vi "PH_PPMA_PowerUnit.PC_StateIgni.vi"(0 "i ref in":refnum<vi>, 3 "Ignitron Status":T1=2 caption="Enabling State" items=["no info", "off/false/out", "on/true/in", "Failure", "Alarm", "Status 1", "Status 2", "Status 3"], 4 "not linked?":bool, 5 "error in (no error)":errorcluster) -> (14 "i ref out":refnum<vi>, 19 "error out":errorcluster)   [LabVIEW 2014, in "PH_PPMA_PowerUnit.lvlib"]
doc: "This VI writes the Ignitron Tag values to own attributes, calculates the state of the device and sets the GUI object."
uses:
  PH_PPMA_PowerUnit.lvlib
  PH_Basics/PH_StatusHandler/PH_StatusHandler.Status.ctl
  PH_Basics/PH_Common/PH_Common.lvlib
  PH_Devices/PH_Beckhoff_PP_PU/PH_Beckhoff_PP_PU.lvlib
  PH_Basics/PH_PowerUnit_BaseClass/PH_PowerUnit_BaseClass.lvlib
  PH_Basics/PH_StatusHandler/PH_StatusHandler.lvlib
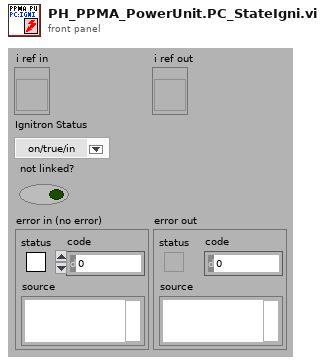
[diagram p1: front panel]
types:
  T1 = typedef "PH_StatusHandler.lvlib/PH_StatusHandler.Status.ctl" = i16
  T2 = typedef "PH_PPMA_PowerUnit.lvlib/PH_PPMA_PowerUnit.i attribute.ctl" = cluster{"GUI Refs":cluster{"Rods":refnum<vi>, "Ignitron":refnum<vi>, "Rossrelais":refnum<vi>, "Set Voltage":refnum<vi>, "PSU":refnum<vi>, "EOC":refnum<vi>, "Trigger":refnum<vi>}, "Rods":T3, "PSU":T4, "Ross Relais":T5, "Ignitron":T6, "Trigger":cluster{"State Device":T1, "linked?":bool}, "Timing Settings":cluster{"Prdc Fast?":bool, "Default Value Periodic Interval":i32, "Mercury on since":dbl, "Warm up Time Mercury [s]":dbl}, "Set Voltage [V]":dbl}
  T3 = typedef "PH_PPMA_PowerUnit.lvlib/PH_PPMA_PowerUnit.Rods Attributes.ctl" = cluster{"Instancename":string, "Device Status":T1, "linked?":bool}
  T4 = typedef "PH_PP_Common.lvlib/PH_PP_Common.PSU Attributes.ctl" = cluster{"lower limit [V]":dbl, "upper limit [V]":dbl, "Voltage set":bool, "State Device":T1, "linked?":bool}
  T5 = typedef "PH_PP_Common.lvlib/PH_PP_Common.Ross Relais Attributes.ctl" = cluster{"State Device":T1, "linked?":bool}
  T6 = typedef "PH_PP_Common.lvlib/PH_PP_Common.Ignitron Attributes.ctl" = cluster{"State Device":T1, "linked?":bool}
  T7 = typedef "PH_PowerUnit_BaseClass.lvlib/PH_PowerUnit_BaseClass.i attribute.ctl" = cluster{"Constructor finished":bool, "PU":cluster{"In use":bool, "Service ID in use":i32, "GUI Ref":refnum<vi>}, "Enabling":cluster{"State":T8, "GUI Ref":refnum<vi>}, "Timing":cluster{"Last Shot":dbl, "Time between Shots [Sec]":dbl, "Waiting Time over?":bool, "Service ID Waiting Time":i32, "GUI Ref":refnum<vi>, "Instance":cluster{"Status":T1, "linked?":bool, "GUI Ref":refnum<vi>}}, "Sequencer":cluster{"SM State":string, "GUI Ref":refnum<vi>, "linked":bool}, "Subscribed Trendmssgs":cluster{"Tagname":string, "Status":T1, "linked?":bool, "Shot Condition":T1, "GUI Ref":refnum<vi>}[], "PP PU":T9, "Default Voltage (V)":dbl, "GUI Refs":T10, "PSDB data":cluster{"Shot Voltage [V]":dbl, "State TO SM":T11, "Write 2 early":bool}, "State TO SM":T11}
  T8 = typedef "PH_SystemInformation.lvlib/PH_SystemInformationEnabling State.ctl" = i32
  T9 = typedef "PH_PP_Common.lvlib/PH_PP_Common.PUs.ctl" = enum16{"no Info", "PA-19mm-1", "PA-19mm-2", "PA-45mm-PILC", "PA-45mm-MAIN", "MA-PU-1", "MA-PU-2", "MA-PU-3", "MA-PU-4", "MA-PU-5", "MA-PU-6", "MA-FR", "MA-PILC", "PA-45mm-DP"}
  T10 = typedef "PH_PowerUnit_BaseClass.lvlib/PH_PowerUnit_BaseClass.GUI Refs.ctl" = cluster{"Delete Inst":refnum<vi>, "State TO SM":refnum<vi>, "State SM":refnum<vi>, "Fire":refnum<vi>}
  T11 = typedef "PH_PowerUnit_BaseClass.lvlib/PH_PowerUnit_BaseClass.SM States.ctl" = enum16{".", "Stand by", "Switch PU on", "Configure", "Set Default Voltage", "Set STANDBY", "Set READY", "Wait for Shot Cmd", "Open Dump Rods", "Open Ross Relais", "Close Ross Relais", "Switch PSU on", "Switch PSU off", "Charge", "Switch GD Channel on", "Close Dump Rods", "Rods-TO", "RR-TO", "PSU-TO", "Trigger-TO"}
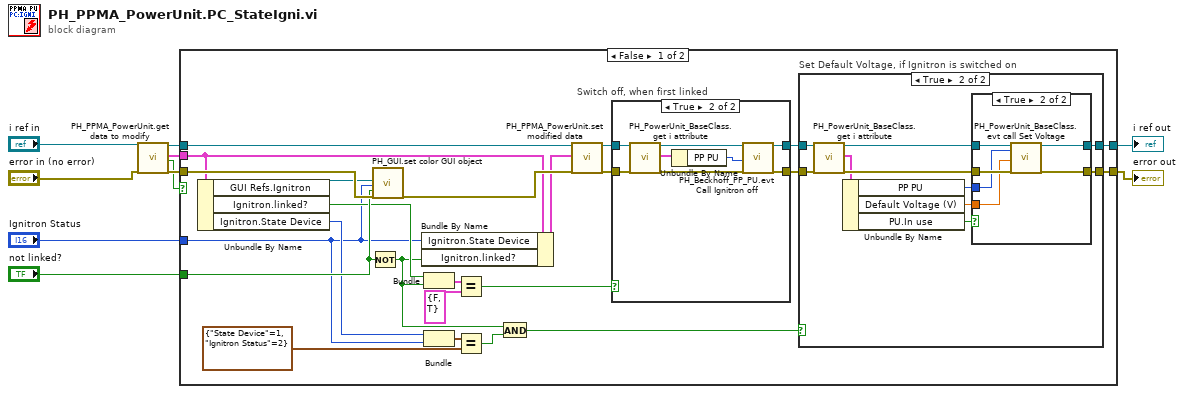
[diagram p0: block diagram]
diagram:
  n1 = call "PH_PPMA_PowerUnit.get data to modify.vi"("i ref in"="i ref in", "error in (no error)"="error in (no error)") -> ("i ref out"=w10:refnum<vi>, "i attribute"=w8:T2, "timed out"=w7:bool, "error out"=w9:errorcluster)  [unwired: 14 in]
  n2 = case shown="False" w7 {
    tunnel: w10 -> [w34 w66]
    tunnel: [w21 w66] -> w4
    tunnel: w9 -> [w33 w65]
    tunnel: [w19 w65] -> w3
    tunnel: w8 -> [w29 _]
    tunnel: "Ignitron Status" -> [w16 _]
    tunnel: "not linked?" -> [w28 _]
    frame False {
      n3 = Unbundle By Name(w29) -> ("GUI Refs.Ignitron"=w30:refnum<vi>, "Ignitron.linked?"=w27:bool, "Ignitron.State Device"=w17:T1)
      n4 = Not(x=w28) -> (.not. x?=w11:bool)
      n5 = call "PH_GUI.set color GUI object.vi"("GUI object Ref"=w30, "State"=w16, "Blinking? (false)"=w28, "error in (no error)"=w33) -> ("error out"=w32:errorcluster)  [unwired: 15 in]
      n6 = Bundle By Name(cluster=w29, "Ignitron.State Device"=w16, "Ignitron.linked?"=w11) -> (w31:T2)
      n7 = Bundle("linked?"=w27, w11) -> (w26:cluster{"linked?":bool, bool})  [unwired: 1 in]
      n8 = Bundle("State Device"=w17, "Ignitron Status"=w16) -> (w15:cluster{"State Device":T1, "Ignitron Status":T1})  [unwired: 1 in]
      n9 = Equal?(x=w26, y=cluster{"linked?":bool, bool} {"linked?"=FALSE, TRUE}) -> (x = y?=w22:bool)
      n10 = Equal?(x=w15, y=cluster{"State Device":T1, "Ignitron Status":T1} {"State Device"=1, "Ignitron Status"=2}) -> (x = y?=w13:bool)
      n11 = And(x=w11, y=w13) -> (x .and. y?=w12:bool)
      n12 = call "PH_PPMA_PowerUnit.set modified data.vi"("i ref in"=w34, "i attribute"=w31, "error in (no error)"=w32) -> ("i ref out"=w23:refnum<vi>, "error out"=w24:errorcluster)  [unwired: 15 in]
      n13 = case "Switch off, when first linked" shown="True" w22 {
        tunnel: w24 -> [w55 w57]
        tunnel: [w55 w64] -> w18
        tunnel: w23 -> [w56 w58]
        tunnel: [w56 w63] -> w20
        frame False {
        }
        frame True {
          n14 = call "PH_PowerUnit_BaseClass.get i attribute.vi"("i ref in"=w58, "error in (no error)"=w57) -> ("i ref out"=w61:refnum<vi>, "i attribute"=w60:T7, "error out"=w62:errorcluster)  [unwired: 15 in]
          n15 = Unbundle By Name(w60) -> ("PP PU"=w59:T9)
          n16 = call "PH_Beckhoff_PP_PU.evt Call Ignitron off.vi"("i ref in"=w61, "PU"=w59, "error in"=w62) -> ("i ref out"=w63:refnum<vi>, "error out"=w64:errorcluster)  [unwired: 15 in]
        }
      }
      n17 = case "Set Default Voltage, if Ignitron is switched on" shown="True" w12 {
        tunnel: [w36 w46] -> w21
        tunnel: w20 -> [w36 w40]
        tunnel: [w35 w45] -> w19
        tunnel: w18 -> [w35 w39]
        frame False {
        }
        frame True {
          n18 = call "PH_PowerUnit_BaseClass.get i attribute.vi"("i ref in"=w40, "error in (no error)"=w39) -> ("i ref out"=w43:refnum<vi>, "i attribute"=w42:T7, "error out"=w44:errorcluster)  [unwired: 15 in]
          n19 = Unbundle By Name(w42) -> ("PP PU"=w41:T9, "Default Voltage (V)"=w38:dbl, "PU.In use"=w37:bool)
          n20 = case shown="True" w37 {
            tunnel: [w47 w54] -> w45
            tunnel: [w48 w53] -> w46
            tunnel: w44 -> [w47 w52]
            tunnel: w43 -> [w48 w51]
            tunnel: w41 -> [_ w50]
            tunnel: w38 -> [_ w49]
            frame False {
            }
            frame True {
              n21 = call "PH_PowerUnit_BaseClass.evt call Set Voltage.vi"("i ref in"=w51, "PowerUnit"=w50, "Voltage [V]"=w49, "error in (no error)"=w52) -> ("i ref out"=w53:refnum<vi>, "error out"=w54:errorcluster)  [unwired: 14 in]
            }
          }
        }
      }
    }
    frame True {
    }
  }
  "error out" <- w3
  "i ref out" <- w4
